vi "error_detect.vi"(4 "error in (no error)":errorcluster, 6 "key bit sequence":u8[](array[numeric]), 7 "input bit sequence":u8[](array[numeric])) -> (0 "error out":errorcluster, 3 "bit-error rate":dbl)   [LabVIEW 2013]
panel:
  # "Compute bit-error rate"
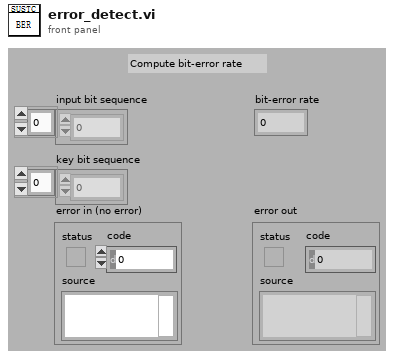
[diagram p1: front panel]
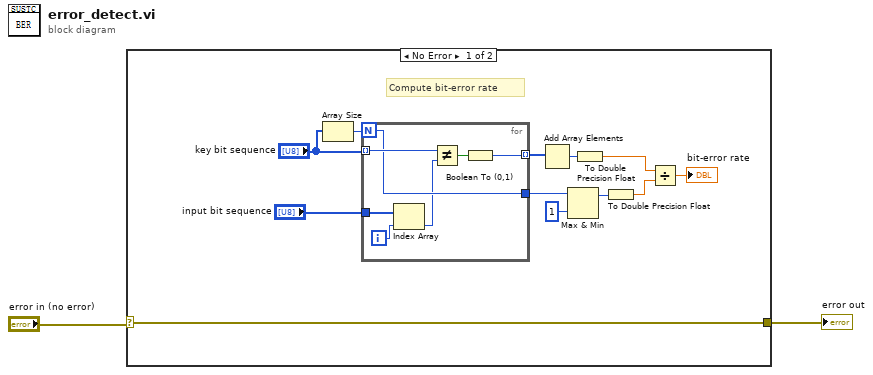
[diagram p0: block diagram]
diagram:
  n1 = case shown="No Error" "error in (no error)" {
    selector: "error in (no error)" -> [w3 w22]
    tunnel: [w3 w22] -> w1
    frame No Error {
      # "Compute bit-error rate"
      n2 = Array Size(array="key bit sequence") -> (size(s)=w14:i32)
      n3 = for {
        N: w14 -> [w18]
        tunnel: "key bit sequence" -> [w20] mode=indexing
        tunnel: "input bit sequence" -> [w17]
        tunnel: [w19] -> w6 mode=indexing
        tunnel: [w18] -> w5
        i -> [w16]
        n4 = Index Array(array=w17, index=w16) -> (element=w15:u8)
        n5 = Not Equal?(x=w20, y=w15) -> (x != y?=w21:bool)
        n6 = Boolean To (0,1)(Boolean=w21) -> (0, 1=w19:i16)
      }
      n7 = Add Array Elements(numeric array=w6) -> (sum=w7:i16)
      n8 = Max & Min(x=w5, y=1) -> (max(x,y)=w9:i32)  [unwired: 1 out]
      n9 = To Double Precision Float(number=w7) -> (double precision float=w10:dbl)
      n10 = To Double Precision Float(number=w9) -> (double precision float=w11:dbl)
      n11 = Divide(x=w10, y=w11) -> (x/y=→"bit-error rate":dbl)
    }
    frame Error {
    }
  }
  "error out" <- w1
